vi "最大值最小值函数.vi"() -> ()   [LabVIEW 2012]
panel:
  out "最小索引":i32
  out "最小值":i32
  out "最大索引":i32
  out "最大值":i32
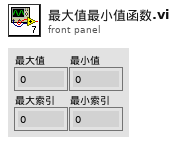
[diagram p1: front panel]
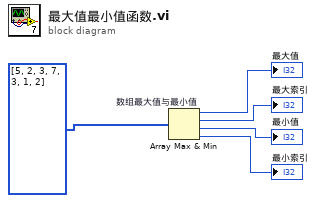
[diagram p0: block diagram]
diagram:
  n1 = Array Max & Min "数组最大值与最小值"(array=i32[] [5, 2, 3, 7, 3, 1, 2]) -> (max value=→"最大值":i32, max index (indices)=→"最大索引":i32, min value=→"最小值":i32, min index (indices)=→"最小索引":i32)
